vi "DidStop.vi"(8 "ErrorArray":errorcluster[](array[cluster]), 10 "Init?":bool, 11 "Bus":refnum<class "Bus.lvclass">) -> (0 "ErrorArray":errorcluster[](array[cluster]), 3 "Bus":refnum<class "Bus.lvclass">)   [LabVIEW 2014, in "Bus_class.lvlib"]
uses:
  Bus_class.lvlib
  Bus.lvclass
  Typedefs/clDidInit.ctl
  Typedefs/clUserEventType.ctl
  <userlib>/NIST/NISTErrorLib/NISTErrorLib.lvlib
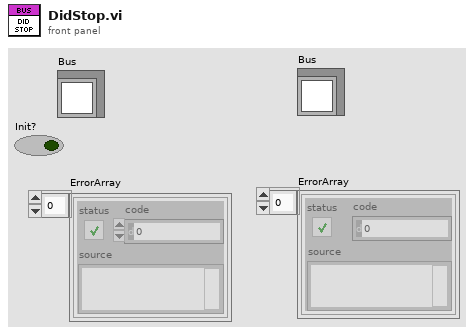
[diagram p1: front panel]
types:
  T1 = typedef "Bus_class.lvlib/clUserEventType.ctl" = cluster{"BusNumber":i8, "Data":variant}
  T2 = typedef "Bus_class.lvlib/clDidInit.ctl" = cluster{"Bus":refnum<vi>, "Init?":bool}
  T3 = typedef "Bus_class.lvlib/clBroadcastEvents.ctl" = cluster{"DidInit":refnum<user-event>, "DidStop":refnum<user-event>}
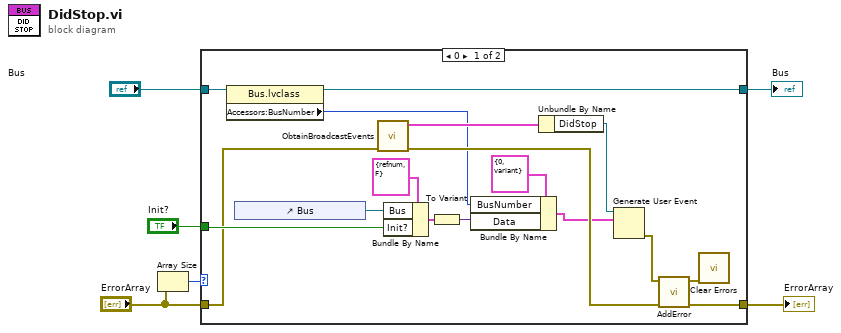
[diagram p0: block diagram]
diagram:
  n1 = Array Size(array="ErrorArray") -> (size(s)=w5:i32)
  n2 = case shown="0" w5 {
    tunnel: "Init?" -> [w20 _]
    tunnel: "ErrorArray" -> [w19 w25]
    tunnel: [w15 w25] -> w3
    tunnel: "Bus" -> [w14 w24]
    tunnel: [w10 w24] -> w1
    frame 0 {
      n3 = property class="Bus.lvclass"(reference=w14) -> (reference out=w10:refnum<class "Bus.lvclass">, "Accessors:BusNumber"=w9:u8)  [unwired: 1 in, 1 out]
      n4 = control-ref of="Bus"() -> (w13:refnum<vi>)
      n5 = call "ObtainBroadcastEvents.vi"("ErrorArray"=w19) -> ("ErrorArray"=w18:errorcluster[], "BusBroadcast"=w23:T3)  [unwired: 9 in]
      n6 = Bundle By Name(cluster=T2 {"Bus"=refnum, "Init?"=FALSE} ("clBusDidInit"), "Bus"=w13, "Init?"=w20) -> (w11:T2)
      n7 = To Variant(anything=w11) -> (Variant=w7:variant)
      n8 = Bundle By Name(cluster=T1 {"BusNumber"=0, "Data"=variant} ("clEventType"), "BusNumber"=w9, "Data"=w7) -> (w8:T1)
      n9 = Unbundle By Name(w23) -> ("DidStop"=w22:refnum<user-event>)
      n10 = Generate User Event(user event=w22, event data cluster=w8) -> (error out=w17:errorcluster)  [unwired: 2 in, 1 out]
      n11 = call <userlib>:"AddError.vi"("ErrorArray"=w18, "error in (no error)"=w17) -> ("ErrorArray"=w15:errorcluster[], "error out"=w16:errorcluster)  [unwired: 8 in]
      n12 = call <vilib>:"Clear Errors.vi"("error in (no error)"=w16) -> ()  [unwired: 5 in, 2 out]
    }
    frame 1, Default {
    }
  }
  "ErrorArray" <- w3
  "Bus" <- w1
